vi "LWXPS_XYLineArcPulseOutputGet.vi"(0 "XPS Reference IN":refnum<k24>, 7 "XY Group name":string, 11 "LabVIEW error IN":errorcluster) -> (3 "XPS Reference OUT":refnum<k24>, 4 "Returned error code":i32, 6 "Start length":dbl, 8 "End length":dbl, 10 "Path length interval":dbl, 14 "LabVIEW error OUT":errorcluster, 15 "XPS Error String":string)   [LabVIEW 2014]
uses:
  D:/XPSQ8_LabView_Library/Development/Source/Dll/Newport.XPS.CommandInterface.dll
  Dll/Newport.XPS.CommandInterface.dll
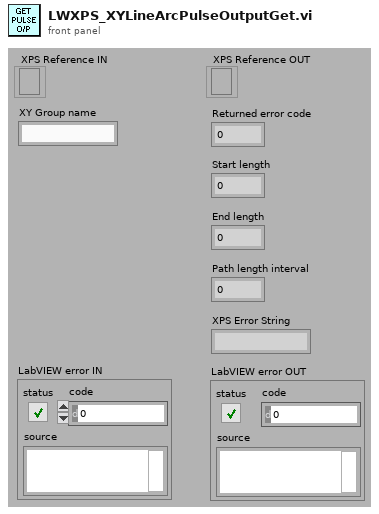
[diagram p1: front panel]
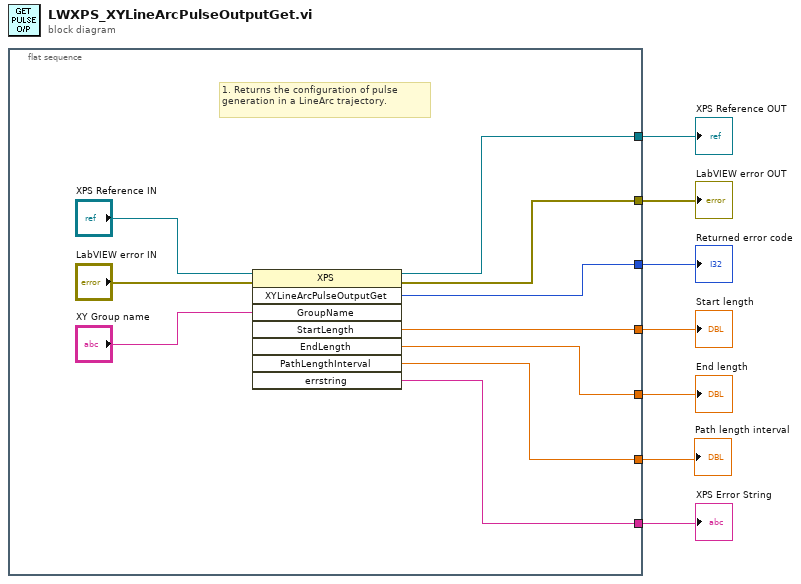
[diagram p0: block diagram]
diagram:
  n1 = flat-sequence {
    tunnel: [w15] -> w7
    tunnel: [w12] -> w6
    tunnel: [w16] -> w5
    tunnel: [w10] -> w3
    tunnel: [w11] -> w4
    tunnel: [w9] -> w1
    tunnel: [w8] -> w2
    frame #0 {
      # "1. Returns the configuration of pulse generation in a LineArc trajectory."
      n2 = invoke class="XPS" method="XYLineArcPulseOutputGet"(reference="XPS Reference IN", error in="LabVIEW error IN", "GroupName"="XY Group name") -> (reference out=w15:refnum<k24>, error out=w12:errorcluster, "XYLineArcPulseOutputGet"=w16:i32, "StartLength"=w10:dbl, "EndLength"=w11:dbl, "PathLengthInterval"=w9:dbl, "errstring"=w8:string)  [unwired: 5 in, 1 out]
    }
  }
  "XPS Error String" <- w2
  "XPS Reference OUT" <- w7
  "LabVIEW error OUT" <- w6
  "Returned error code" <- w5
  "End length" <- w4
  "Start length" <- w3
  "Path length interval" <- w1
